vi "String_verknuepfen.vi"(8 "error in (no error)":errorcluster caption="Fehler (Eingang, kein Fehler)", 11 "Order":string) -> (0 "error out":errorcluster caption="Fehler (Ausgang)", 3 "Verknüpfter String":string)   [LabVIEW 2020, in "Linearisierung v2.lvlib" / "Gasteiler.lvlib" / "HovaCAL_Interface.lvlib" / "KGN.lvlib"]
uses:
  KGN.lvlib
panel:
  in  "Zieladresse":string="FF"
  in  "Quelladresse":string="00"
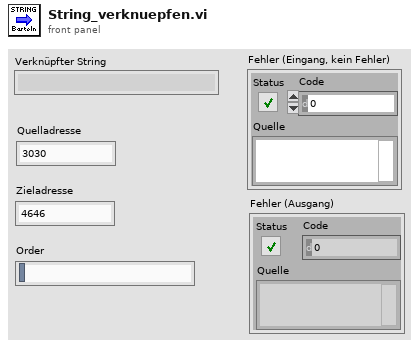
[diagram p1: front panel]
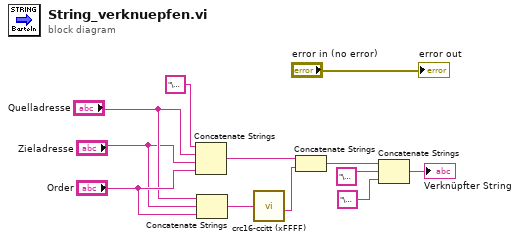
[diagram p0: block diagram]
diagram:
  n1 = Concatenate Strings("\u0002", "Quelladresse", "Zieladresse", "Order") -> (w5:string)
  n2 = Concatenate Strings("Quelladresse", "Zieladresse", "Order") -> (w2:string)
  n3 = call "crc16-ccitt (xFFFF).vi"("Message"=w2) -> ("Hex-Integer-String"=w3:string)  [unwired: 8 in, 2 out]
  n4 = Concatenate Strings(w5, w3) -> (w8:string)
  n5 = Concatenate Strings(w8, "\u0003", "\u0006" ("String")) -> (→"Verknüpfter String":string)
  "error out" <- "error in (no error)"
